vi "Drive_Utils_XYtoDistanceAngle.vi"(3 "error in":errorcluster, 4 "Y":dbl, 5 "X":dbl) -> (0 "error out":errorcluster, 1 "Angle (rad)":dbl, 2 "Distance":dbl)   [LabVIEW 2009, in "Drive.lvlib" / "Drive_Utils.lvlib"]
doc: "Transforms XY coordinates to polar coordinates (distance and angle)"
uses:
  Drive_Utils.lvlib
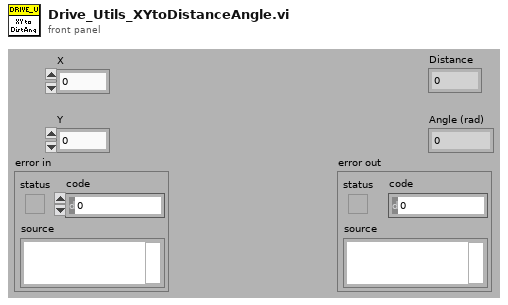
[diagram p1: front panel]
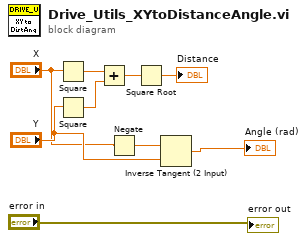
[diagram p0: block diagram]
diagram:
  n1 = Square(x="X") -> (x^2=w7:dbl)
  n2 = Square(x="Y") -> (x^2=w6:dbl)
  n3 = Add(x=w7, y=w6) -> (x+y=w8:dbl)
  n4 = Negate(x="X") -> (-x=w3:dbl)
  n5 = Square Root(x=w8) -> (sqrt(x)=→"Distance":dbl)
  n6 = Inverse Tangent (2 Input)(1:"Y", 2:w3) -> (0:→"Angle (rad)":dbl)
  "error out" <- "error in"
